vi "ReplaceSelf.vi"(0 "XRef":T17, 1 "Terms":T14, 2 "Diagram":T13, 3 "State In":T5) -> (14 "Replace Self?":T4, 15 "Reply":T2, 16 "Fatal Error Out":T1)   [LabVIEW 2021, in "myRIO DO N Samples Open.xnode"]
uses:
  <vilib>/myRIO/Instrument Drivers/Onboard IO/DO Block/vis/myRIO DO N Samples Open.xnode
  <vilib>/XNodeSupport/XNodeXNodeRef.ctl
  <vilib>/XNodeSupport/XNodeTermIDPairs.ctl
  <vilib>/XNodeSupport/XNodeTermIDPair.ctl
  <vilib>/XNodeSupport/XNodeTermRef.ctl
  <vilib>/XNodeSupport/XNodeString.ctl
  <vilib>/XNodeSupport/XNodeTopLevelDiagramRef.ctl
  <vilib>/myRIO/Instrument Drivers/Onboard IO/DO Block/vis/State.ctl
  <vilib>/myRIO/Common/Instrument Driver Framework/Utilities/typedefs/myRIOXPeripheral.ctl
  <vilib>/XNodeSupport/XNodeTerm4Array.ctl
  <vilib>/XNodeSupport/XNodeTerm4.ctl
  <vilib>/XNodeSupport/XNodeVariant.ctl
  <vilib>/XNodeSupport/XNodeRect32.ctl
  <vilib>/XNodeSupport/XNodeInt.ctl
  <vilib>/XNodeSupport/XNodeBool.ctl
  <vilib>/XNodeSupport/XNodeTermDirection.ctl
  <vilib>/XNodeSupport/XNodeStringArray.ctl
  <vilib>/XNodeSupport/XNodeErrorCluster.ctl
  <vilib>/myRIO/Common/Instrument Driver Framework/Utilities/vis/myRIOXGlobal.vi
  <vilib>/XNodeSupport/NI_XNodeSupport.lvlib
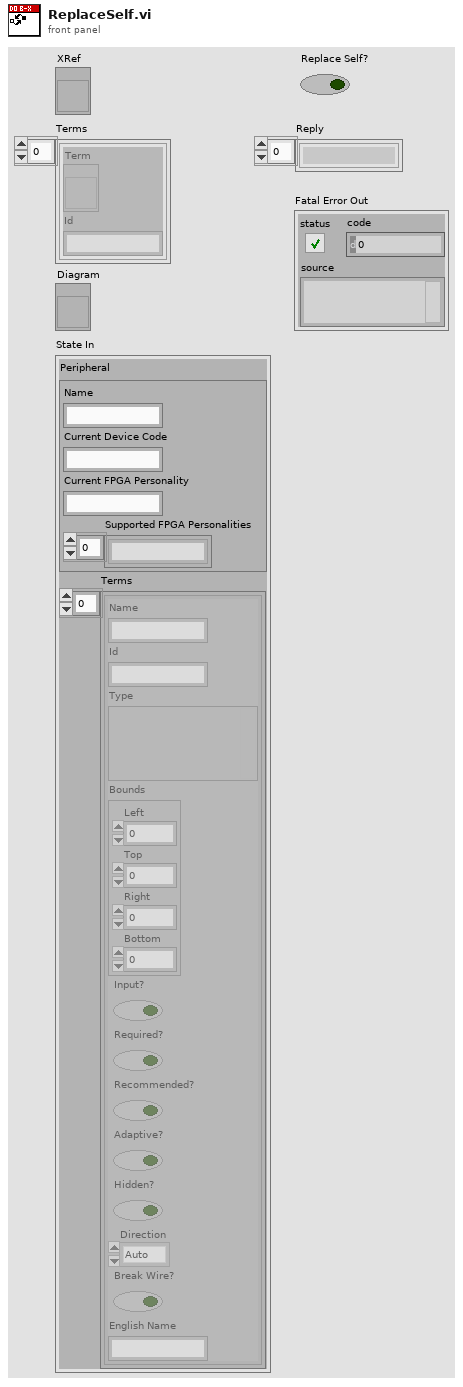
[diagram p1: front panel]
types:
  T1 = typedef "NI_XNodeSupport.lvlib/XNodeErrorCluster.ctl" = errorcluster
  T2 = typedef "NI_XNodeSupport.lvlib/XNodeStringArray.ctl" = T3[]
  T3 = typedef "NI_XNodeSupport.lvlib/XNodeString.ctl" = string
  T4 = typedef "NI_XNodeSupport.lvlib/XNodeBool.ctl" = bool
  T5 = typedef "myRIO DO N Samples Open.xnode/State.ctl" = cluster{"Peripheral":T6, "Terms":T7}
  T6 = typedef "myRIOXPeripheral.ctl" = cluster{"Name":string, "Current Device Code":string, "Current FPGA Personality":string, "Supported FPGA Personalities":string[]}
  T7 = typedef "NI_XNodeSupport.lvlib/XNodeTerm4Array.ctl" = T8[]
  T8 = typedef "NI_XNodeSupport.lvlib/XNodeTerm4.ctl" = cluster{"Name":T3, "Id":T3, "Type":T9, "Bounds":T10, "Input?":T4, "Required?":T4, "Recommended?":T4, "Adaptive?":T4, "Hidden?":T4, "Direction":T12, "Break Wire?":T4, "English Name":T3}
  T9 = typedef "NI_XNodeSupport.lvlib/XNodeVariant.ctl" = variant
  T10 = typedef "NI_XNodeSupport.lvlib/XNodeRect32.ctl" = cluster{"Left":T11, "Top":T11, "Right":T11, "Bottom":T11}
  T11 = typedef "NI_XNodeSupport.lvlib/XNodeInt.ctl" = i32
  T12 = typedef "NI_XNodeSupport.lvlib/XNodeTermDirection.ctl" = enum32{"Auto", "Up", "Down", "Left", "Right", "Center"}
  T13 = typedef "NI_XNodeSupport.lvlib/XNodeTopLevelDiagramRef.ctl" = refnum<vi>
  T14 = typedef "NI_XNodeSupport.lvlib/XNodeTermIDPairs.ctl" = T15[]
  T15 = typedef "NI_XNodeSupport.lvlib/XNodeTermIDPair.ctl" = cluster{"Term":T16, "Id":T3}
  T16 = typedef "NI_XNodeSupport.lvlib/XNodeTermRef.ctl" = refnum<vi>
  T17 = typedef "NI_XNodeSupport.lvlib/XNodeXNodeRef.ctl" = refnum<vi>
  T18 = typedef "NI_XNodeSupport.lvlib/XNodeImage.ctl" = picture
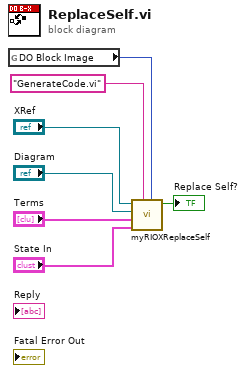
[diagram p0: block diagram]
diagram:
  n1 = global read "myRIOXGlobal.vi" "DO Block Image"() -> (w1:T18)
  n2 = call <vilib>:"myRIOXReplaceSelf.vi"("ICON Image"=w1, "Generate Code VI Name"="GenerateCode.vi", "State In"="State In", "Terms"="Terms", "Diagram"="Diagram", "XRef"="XRef") -> ("Replace Self?"=→"Replace Self?":T4)  [unwired: 5 in]
